vi "SngJntArmSim_Rkf45_Func.vi"(9 "U":T1, 10 "X":T1, 11 "Variant":variant) -> (0 "Error":bool, 3 "NewX":T1)   [LabVIEW 2019, in "Trajectory_Library.lvlib"]
doc: "Custom function to calculate the newX used for integrating to get updated HatX \n\n\nInputs:\n - Variant -- extra data used by function\n for this function, the extra data is; Matrix A, Matrix B, Arm length, Simulator gravity flag.\n - X - X matrix\n - U - U matrix\n\nOutputs:\n - NewX -- X value as a function of (X, U, extra data)\n - error -- If TRUE, an error occured."
uses:
  Trajectory_Library.lvlib
  <vilib>/Analysis/Matrix/Datatypes/RealMatrix.ctl
  <vilib>/Analysis/Matrix/NI_Matrix.lvlib
  <vilib>/Analysis/NI_AALBase.lvlib
  <vilib>/Analysis/baseanly.llb/Real A x B.vi
  <vilib>/Analysis/Matrix/Numeric/Add/Add - RM,RM.vi
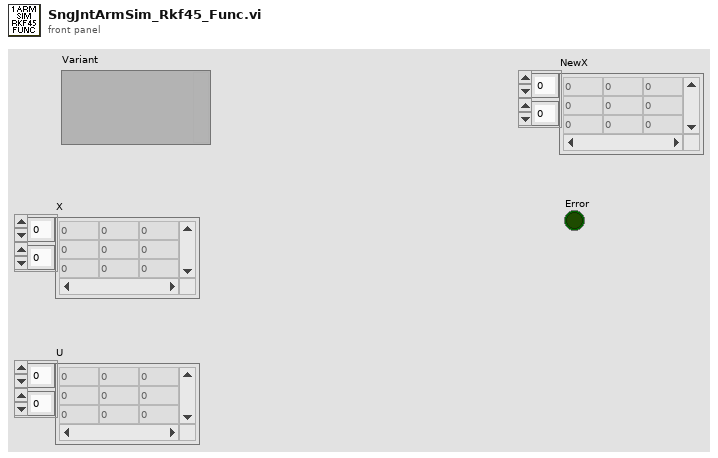
[diagram p1: front panel]
types:
  T1 = typedef "NI_Matrix.lvlib/RealMatrix.ctl" = dbl[][]
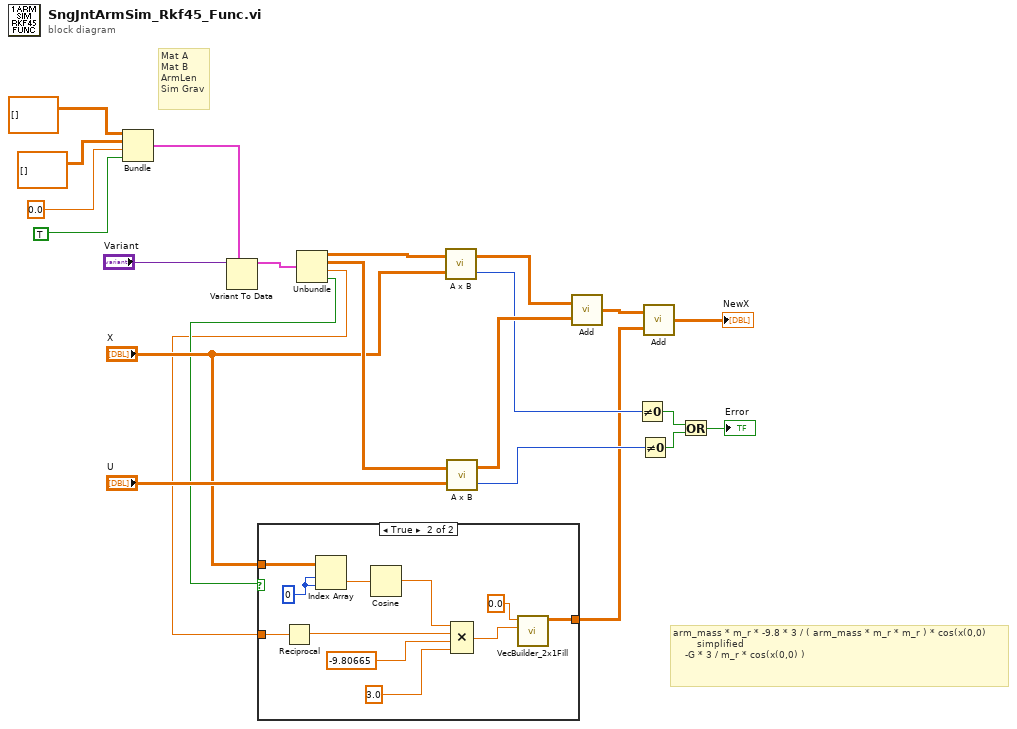
[diagram p0: block diagram]
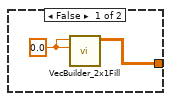
[diagram p2: hidden frame]
diagram:
  # "arm_mass * m_r * -9.8 * 3 / ( arm_mass * m_r * m_r ) * cos(x(0,0)\n        simplified\n    -G * 3 / m_r * cos(x(0,0) )"
  # "Mat A\nMat B\nArmLen\nSim Grav"
  n1 = Bundle("matrix"=T1 [], "matrix"=T1 [], 0.0, TRUE) -> (w20:cluster{"matrix":T1, "matrix":T1, dbl, bool})  [unwired: 1 in]
  n2 = Variant To Data(type=w20, Variant="Variant") -> (data=w19:cluster{"matrix":T1, "matrix":T1, dbl, bool})  [unwired: 1 in, 1 out]
  n3 = Unbundle(w19) -> ("matrix"=w11:T1, "matrix"=w10:T1, w1:dbl, w2:bool)
  n4 = case shown="True" w2 {
    tunnel: [w24 w35] -> w6
    tunnel: "X" -> [_ w33]
    tunnel: w1 -> [_ w31]
    frame False {
      w25 = 0.0 ("R0")
      n5 = call "VecBuilder_2x1Fill.vi"("R1"=w25, "R0"=w25) -> ("output matrix"=w24:T1)  [unwired: 9 in]
    }
    frame True {
      w34 = 0 ("index (row)")
      n6 = Reciprocal(x=w31) -> (1/x=w29:dbl)
      n7 = Index Array(array=w33, index (row)=w34, index (col)=w34) -> (element=w32:dbl)
      n8 = Cosine(x=w32) -> (cos(x)=w30:dbl)
      n9 = Compound Arithmetic op=MULTIPLY(w30, w29, -9.80665 ("R1"), 3.0 ("R1")) -> (w26:dbl)
      n10 = call "VecBuilder_2x1Fill.vi"("R1"=w26, "R0"=0.0) -> ("output matrix"=w35:T1)  [unwired: 9 in]
    }
  }
  n11 = call-poly <vilib>:"A x B.vi"("B"="X", "A"=w11) -> ("error"=w13:i32, "A x B"=w18:T1)
  n12 = call-poly <vilib>:"A x B.vi"("B"="U", "A"=w10) -> ("error"=w12:i32, "A x B"=w17:T1)
  n13 = call-poly <vilib>:"Add.vi"("Real Matrix B"=w17, "Real Matrix A"=w18) -> ("A + B"=w16:T1)
  n14 = Not Equal To 0?(x=w13) -> (x != 0?=w15:bool)
  n15 = Not Equal To 0?(x=w12) -> (x != 0?=w14:bool)
  n16 = call-poly <vilib>:"Add.vi"("Real Matrix B"=w6, "Real Matrix A"=w16) -> ("A + B"=→"NewX":T1)
  n17 = Or(x=w15, y=w14) -> (x .or. y?=→"Error":bool)
